vi "Autozero.vi"(0 "Vmin (V)":dbl, 2 "Enable":bool, 3 "Max Gain":bool) -> ()   [LabVIEW 2025]
panel:
  # "Adjusts offset to eliminate\npedestal drift"
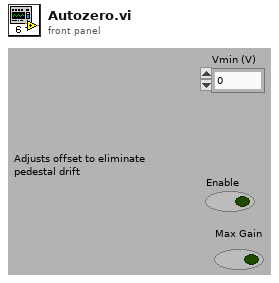
[diagram p1: front panel]
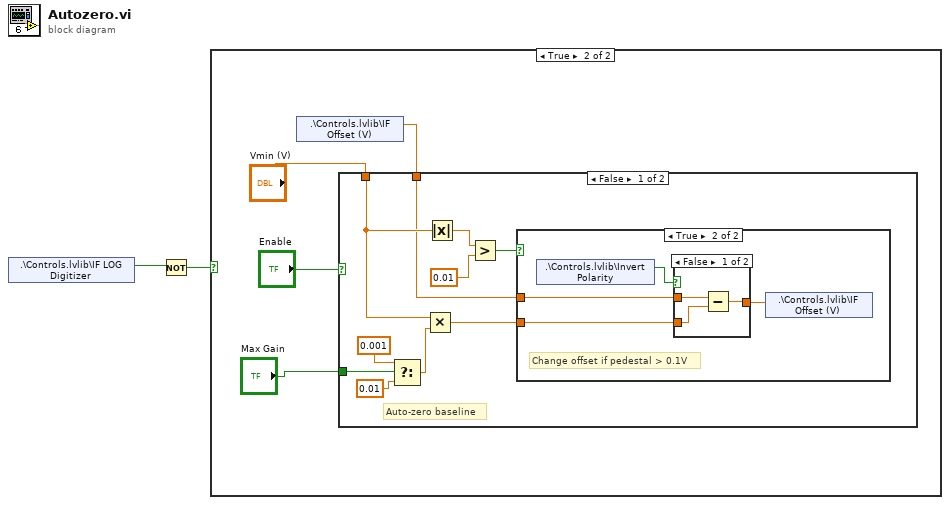
[diagram p0: block diagram]
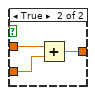
[diagram p4: hidden frame]
diagram:
  n1 = shared-variable ".\\Controls.lvlib\\IF LOG Digitizer"() -> (w1:bool)  [unwired: 1 in, 1 out]
  n2 = Not(x=w1) -> (.not. x?=w2:bool)
  n3 = case shown="True" w2 {
    frame False {
    }
    frame True {
      n4 = shared-variable ".\\Controls.lvlib\\IF Offset (V)"() -> (w3:dbl)  [unwired: 1 in, 1 out]
      n5 = case shown="False" "Enable" {
        tunnel: "Vmin (V)" -> [w14 _]
        tunnel: w3 -> [w13 _]
        tunnel: "Max Gain" -> [w11 _]
        frame False {
          # "Auto-zero baseline"
          n6 = Select(t=0.001, s=w11, f=0.01) -> (s? t:f=w10:dbl)
          n7 = Multiply(x=w14, y=w10) -> (x*y=w12:dbl)
          n8 = Absolute Value(x=w14) -> (abs(x)=w15:dbl)
          n9 = Greater?(x=w15, y=0.01) -> (0:w7:bool)
          n10 = case shown="True" w7 {
            tunnel: w12 -> [_ w20]
            tunnel: w13 -> [_ w19]
            frame False {
            }
            frame True {
              # "Change offset if pedestal > 0.1V"
              n11 = shared-variable ".\\Controls.lvlib\\Invert Polarity"() -> (w18:bool)  [unwired: 1 in, 1 out]
              n12 = case shown="False" w18 {
                tunnel: w20 -> [w21 w26]
                tunnel: w19 -> [w22 w25]
                tunnel: [w23 w24] -> w17
                frame False {
                  n13 = Subtract(x=w22, y=w21) -> (x-y=w23:dbl)
                }
                frame True {
                  n14 = Add(x=w25, y=w26) -> (x+y=w24:dbl)
                }
              }
              n15 = shared-variable ".\\Controls.lvlib\\IF Offset (V)"(w17) -> ()  [unwired: 1 in, 1 out]
            }
          }
        }
        frame True {
        }
      }
    }
  }
